vi "Lift to can.vi"(8 "Desired Height":dbl, 9 "Refnum in":refnum<k33>) -> (3 "Refnum out":refnum<k33>)   [LabVIEW 2014]
uses:
  Co-Pilot_game_control.ctl
  Lifter Hights.vi
  encoderData.vi
panel:
  in  "auton height":T1={"Left_Intake"=0.0, "Right_Intake"=0.0, "Time Stamp"=0, "Command"=enum."Noop", "ToggleCollector"=FALSE, "ManualLift"=0.0, "Top_Limit_Switch"=FALSE, "Bottom_Limit_Switch "=FALSE, "LifterOverride"=FALSE, "AutoLift"=16, "Toggle Auto Lifter"=FALSE, "Activate HP indexer"=FALSE}
  out "error out":errorcluster
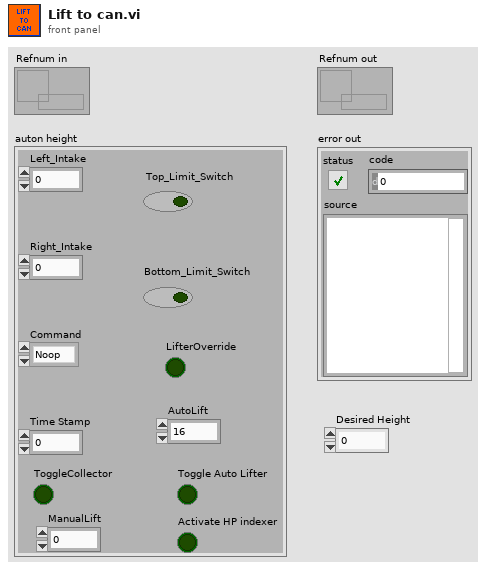
[diagram p1: front panel]
types:
  T1 = typedef "Co-Pilot_game_control.ctl" = cluster{"Left_Intake":dbl, "Right_Intake":dbl, "Time Stamp":u32, "Command":enum16{"Noop", "Flagged"}, "ToggleCollector":bool, "ManualLift":dbl, "Top_Limit_Switch":bool, "Bottom_Limit_Switch ":bool, "LifterOverride":bool, "AutoLift":i32, "Toggle Auto Lifter":bool, "Activate HP indexer":bool}
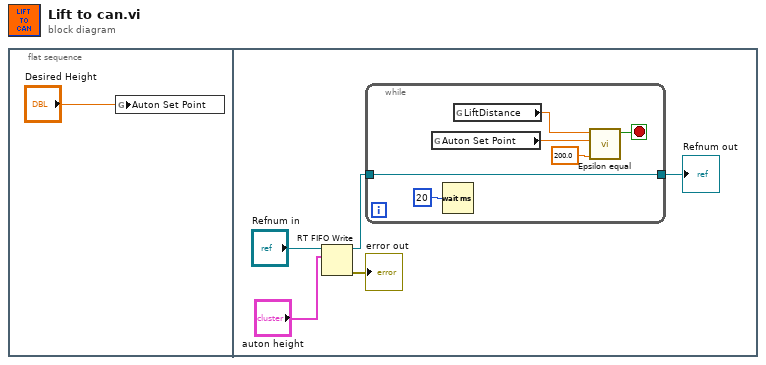
[diagram p0: block diagram]
diagram:
  n1 = flat-sequence {
    frame #0 {
      n2 = global write "Lifter Hights.vi" "Auton Set Point"("Desired Height") -> ()
    }
    frame #1 {
      n3 = RT FIFO Write(0:"Refnum in", 1:"auton height") -> (8:w5:refnum<k33>, 11:→"error out":errorcluster)  [unwired: 3 in, 2 out]
      n4 = while {
        tunnel: w5 -> [w7]
        tunnel: [w7] -> w6
        stop <- w12 stop-if-true
        n5 = global read "Lifter Hights.vi" "Auton Set Point"() -> (w10:dbl)
        n6 = Wait (ms)(milliseconds to wait=u32 20) -> ()  [unwired: 1 out]
        n7 = global read "encoderData.vi" "LiftDistance"() -> (w11:dbl)
        n8 = call "Epsilon equal.vi"("Epsilon"=200.0, "Value2"=w10, "Value1"=w11) -> ("Boolean"=w12:bool)  [unwired: 8 in]
      }
      "Refnum out" <- w6
    }
  }
